vi "InitRGBStudentVersion.vi"(2 "error in (no error)":errorcluster) -> (0 "error out":errorcluster)   [LabVIEW 2016]
uses:
  <vilib>/myRIO/Instrument Drivers/Onboard IO/I2C/typedefs/I2C Transfer Rate.ctl
  <vilib>/myRIO/Instrument Drivers/Onboard IO/I2C/I2C.lvlib
  <vilib>/myRIO/Instrument Drivers/Onboard IO/I2C/typedefs/I2C User Configuration.ctl
  <vilib>/myRIO/Instrument Drivers/Onboard IO/I2C/typedefs/I2C Configuration.ctl
  <vilib>/myRIO/Common/Instrument Driver Framework/myRIO v1.0/I2C/typedefs/I2C Channels Enum.ctl
  <vilib>/myRIO/Common/Instrument Driver Framework/Utilities/typedefs/Generic FPGA Reference.ctl
  <vilib>/myRIO/Common/Instrument Driver Framework/Utilities/typedefs/myRIO v1.0 Reference.ctl
  <vilib>/myRIO/Common/Instrument Driver Framework/Utilities/typedefs/Hardware Version Enum.ctl
  <vilib>/myRIO/Common/Instrument Driver Framework/Utilities/typedefs/myRIO Generic Hardware Reference.ctl
  <vilib>/myRIO/Instrument Drivers/Onboard IO/I2C/typedefs/I2C Reference.ctl
  <vilib>/myRIO/Instrument Drivers/Onboard IO/I2C/vis/Configure.vi
  <vilib>/userdefined/High Color/nirio_resource_hc.ctl
  <vilib>/myRIO/Common/Instrument Driver Framework/myRIO v1.0/I2C/vis/myRIO v1.1 Open I2C.vi
  <vilib>/myRIO/Instrument Drivers/Onboard IO/I2C/vis/myRIO I2C Open.xnode
  <vilib>/myRIO/Common/Instrument Driver Framework/Utilities/vis/Is FPGA Ref Available.vi
  <vilib>/myRIO/Express VI/Onboard IO/I2C/I2C Express VI.xnode
  <vilib>/myRIO/Instrument Drivers/Onboard IO/I2C/vis/Write.vi
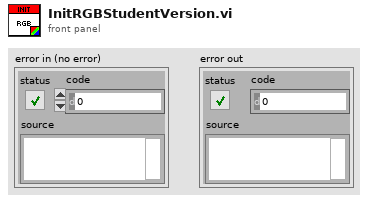
[diagram p1: front panel]
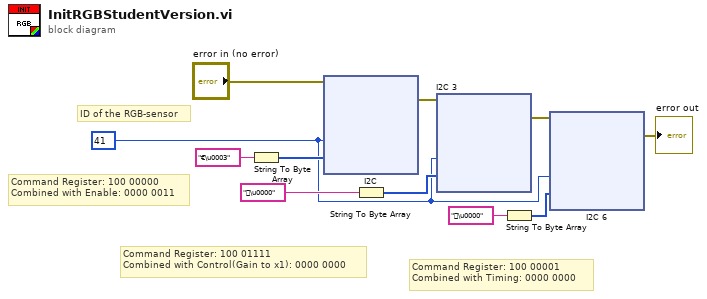
[diagram p0: block diagram]
diagram:
  w5 = 41 ("Numeric")
  # "ID of the RGB-sensor"
  # "Command Register: 100 00000\nCombined with Enable: 0000 0011"
  # "Command Register: 100 01111\nCombined with Control(Gain to x1): 0000 0000"
  # "Command Register: 100 00001\nCombined with Timing: 0000 0000"
  n1 = String To Byte Array(string="€\u0003") -> (unsigned byte array=w8:u8[])
  n2 = xnode "I2C"("Slave Address (7-bit)"=w5, "Bytes to Write"=w8, "error in (no error)"="error in (no error)") -> ("error out"=w4:errorcluster)
  n3 = String To Byte Array(string="\u0000") -> (unsigned byte array=w7:u8[])
  n4 = xnode "I2C 3"("Slave Address (7-bit)"=w5, "Bytes to Write"=w7, "error in (no error)"=w4) -> ("error out"=w3:errorcluster)
  n5 = String To Byte Array(string="\u0000") -> (unsigned byte array=w6:u8[])
  n6 = xnode "I2C 6"("Slave Address (7-bit)"=w5, "Bytes to Write"=w6, "error in (no error)"=w3) -> ("error out"=→"error out":errorcluster)
